vi "Update_Data.vi"(8 "error in (no error)":errorcluster caption="entrée d'erreur (pas d'erreur)", 11 "Firebase AssembledProducts en entrée":refnum<class "Firebase AssembledProducts.lvclass">) -> (0 "error out":errorcluster caption="sortie d'erreur", 3 "Firebase AssembledProducts en sortie":refnum<class "Firebase AssembledProducts.lvclass">)   [LabVIEW 2020, in "Library Instrument & Equipement.lvlib" / "Library FireBase.lvlib" / "Firebase AssembledProducts.lvclass"]
doc: "Create New document\nPlease initialise the following values\n - Name BDD\n - Document\n - API Key"
uses:
  Firebase AssembledProducts.lvclass
  C:/Users/ngarcin/OneDrive - Altyor/Standard TB/Class/Firebase/Source/Firebase Driver/Firebase Driver.lvclass
  Firebase AssembledProducts.lvclass/Firebase AssembledProducts.ctl
  Firebase Altyor/Firebase Altyor.lvclass
  Firebase Driver/Firebase Driver.lvclass
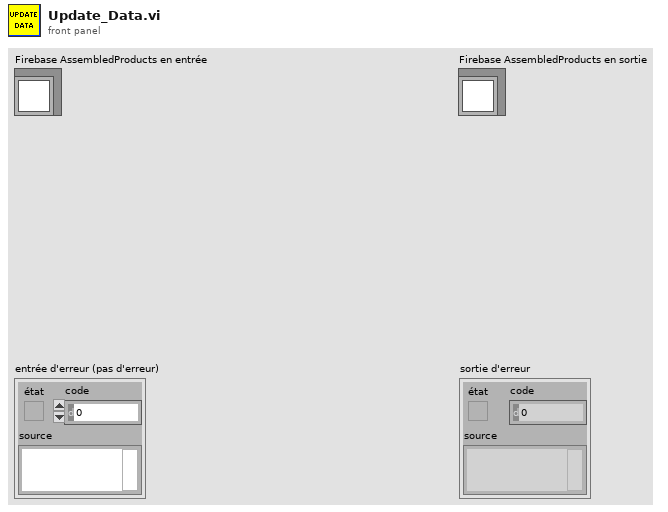
[diagram p1: front panel]
types:
  T1 = cluster{"fields":cluster{"Result":cluster{"booleanValue":bool}, "CreationDate":cluster{"timestampValue":string}, "Batch":cluster{"stringValue":string}, "SerialNumber":cluster{"stringValue":string}, "EndOfProduction":cluster{"timestampValue":string}, "FW_Version":cluster{"mapValue":cluster{"fields":cluster{"Bootloader":cluster{"mapValue":cluster{"fields":cluster{"File_Name":cluster{"stringValue":string}, "Version":cluster{"mapValue":cluster{"fields":cluster{"Major":cluster{"stringValue":string}, "Minor":cluster{"stringValue":string}}}}, "Checksum":cluster{"stringValue":string}}}}, "SoftDevice":cluster{"mapValue":cluster{"fields":cluster{"File_Name":cluster{"stringValue":string}, "Version":cluster{"mapValue":cluster{"fields":cluster{"Major":cluster{"stringValue":string}, "Minor":cluster{"stringValue":string}}}}, "Checksum":cluster{"stringValue":string}}}}, "DFU":cluster{"mapValue":cluster{"fields":cluster{"File_Name":cluster{"stringValue":string}, "Version":cluster{"mapValue":cluster{"fields":cluster{"Major":cluster{"stringValue":string}, "Minor":cluster{"stringValue":string}}}}, "Checksum":cluster{"stringValue":string}}}}}}}, "PartNumber":cluster{"stringValue":string}, "OrderNumber":cluster{"stringValue":string}, "Operator":cluster{"stringValue":string}, "AssembledProductName":cluster{"stringValue":string}}}
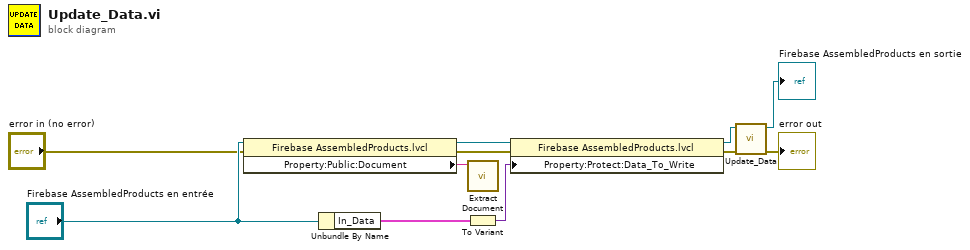
[diagram p0: block diagram]
diagram:
  n1 = property class="Firebase AssembledProducts.lvcl"(reference="Firebase AssembledProducts en entrée", error in="error in (no error)") -> (reference out=w1:refnum<class "Firebase AssembledProducts.lvclass">, error out=w2:errorcluster, "Property:Public:Document"=w7:string)
  n2 = Unbundle By Name("Firebase AssembledProducts en entrée") -> ("In_Data"=w9:T1)
  n3 = call "Extract Document.vi"("Name"=w7) -> ()  [unwired: 9 in, 2 out]
  n4 = To Variant(anything=w9) -> (Variant=w8:variant)
  n5 = property class="Firebase AssembledProducts.lvcl"(reference=w1, error in=w2, "Property:Protect:Data_To_Write"=w8) -> (reference out=w5:refnum<class "Firebase AssembledProducts.lvclass">, error out=w3:errorcluster)
  n6 = call-parent "Update_Data.vi"("error in (no error)"=w3, "Firebase Altyor en entrée"=w5) -> ("error out"=→"error out":errorcluster, "Firebase Altyor en sortie"=→"Firebase AssembledProducts en sortie":refnum<class "Firebase AssembledProducts.lvclass">)  [unwired: 8 in]
